vi "Location_Correction.vi"() -> ()   [LabVIEW 2017]
uses:
  <vilib>/Utility/file.llb/Write Delimited Spreadsheet (DBL).vi
  <vilib>/vision/driver/NI_Vision_Acquisition_Software.lvlib
  <vilib>/vision/NI_Vision_Development_Module.lvlib
panel:
  in  "OK Button":bool
  out "Boolean 2":bool
  out "X":dbl[](array[numeric])
  out "Boolean":bool
  out "Y":dbl[](array[numeric])
  out "選擇範圍 2":T1(plugin-control)
  out "error out":errorcluster
  in  "亮度":cluster{"Min":i32, "Max":i32}(slide)={"Min"=60, "Max"=157} scale=0.0..255.0
  in  "飽和度":cluster{"Min":i32, "Max":i32}(slide)={"Min"=0, "Max"=42} scale=0.0..255.0
  in  "色相":cluster{"Min":i32, "Max":i32}(slide)={"Min"=67, "Max"=120} scale=0.0..255.0
  out "顯示錯誤":errorcluster
  out "影像":T1(plugin-control)
  in  "stop":bool
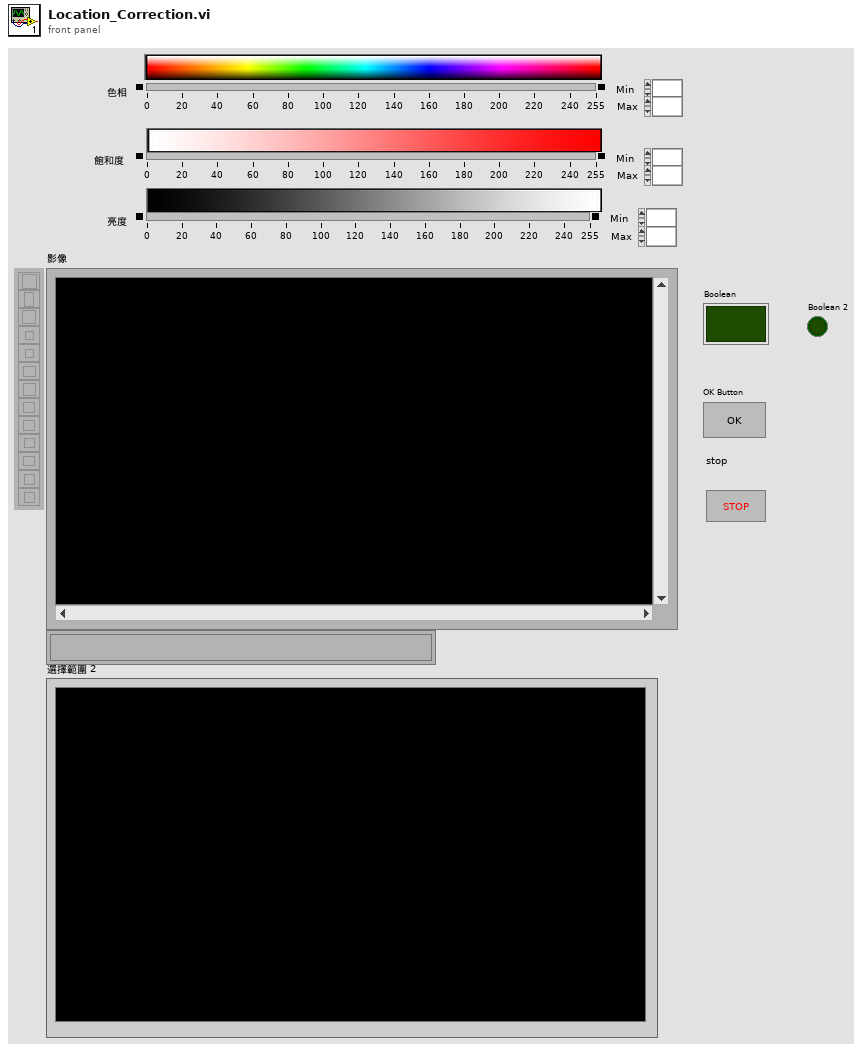
[diagram p1: front panel]
types:
  T1 = typedef "IMAQ Image.ctl" = refnum<image>
  T2 = typedef "Image Type" = u32
  T3 = cluster{"Type":u32, "Version":u32, "Flags":u32, "SerialNumberHigh":u32, "SerialNumberLow":u32, "BusType":u32, "InterfaceName":string, "VendorName":string, "ModelName":string, "CameraFileName":string, "CameraAttributeURL":string}[]
  T4 = cluster{"Type":u32, "Version":u32, "Flags":u32, "SerialNumberHigh":u32, "SerialNumberLow":u32, "BusType":u32, "InterfaceName":string, "VendorName":string, "ModelName":string, "CameraFileName":string, "CameraAttributeURL":string}
  T5 = typedef "IMAQdx.ctl" = refnum<k21>
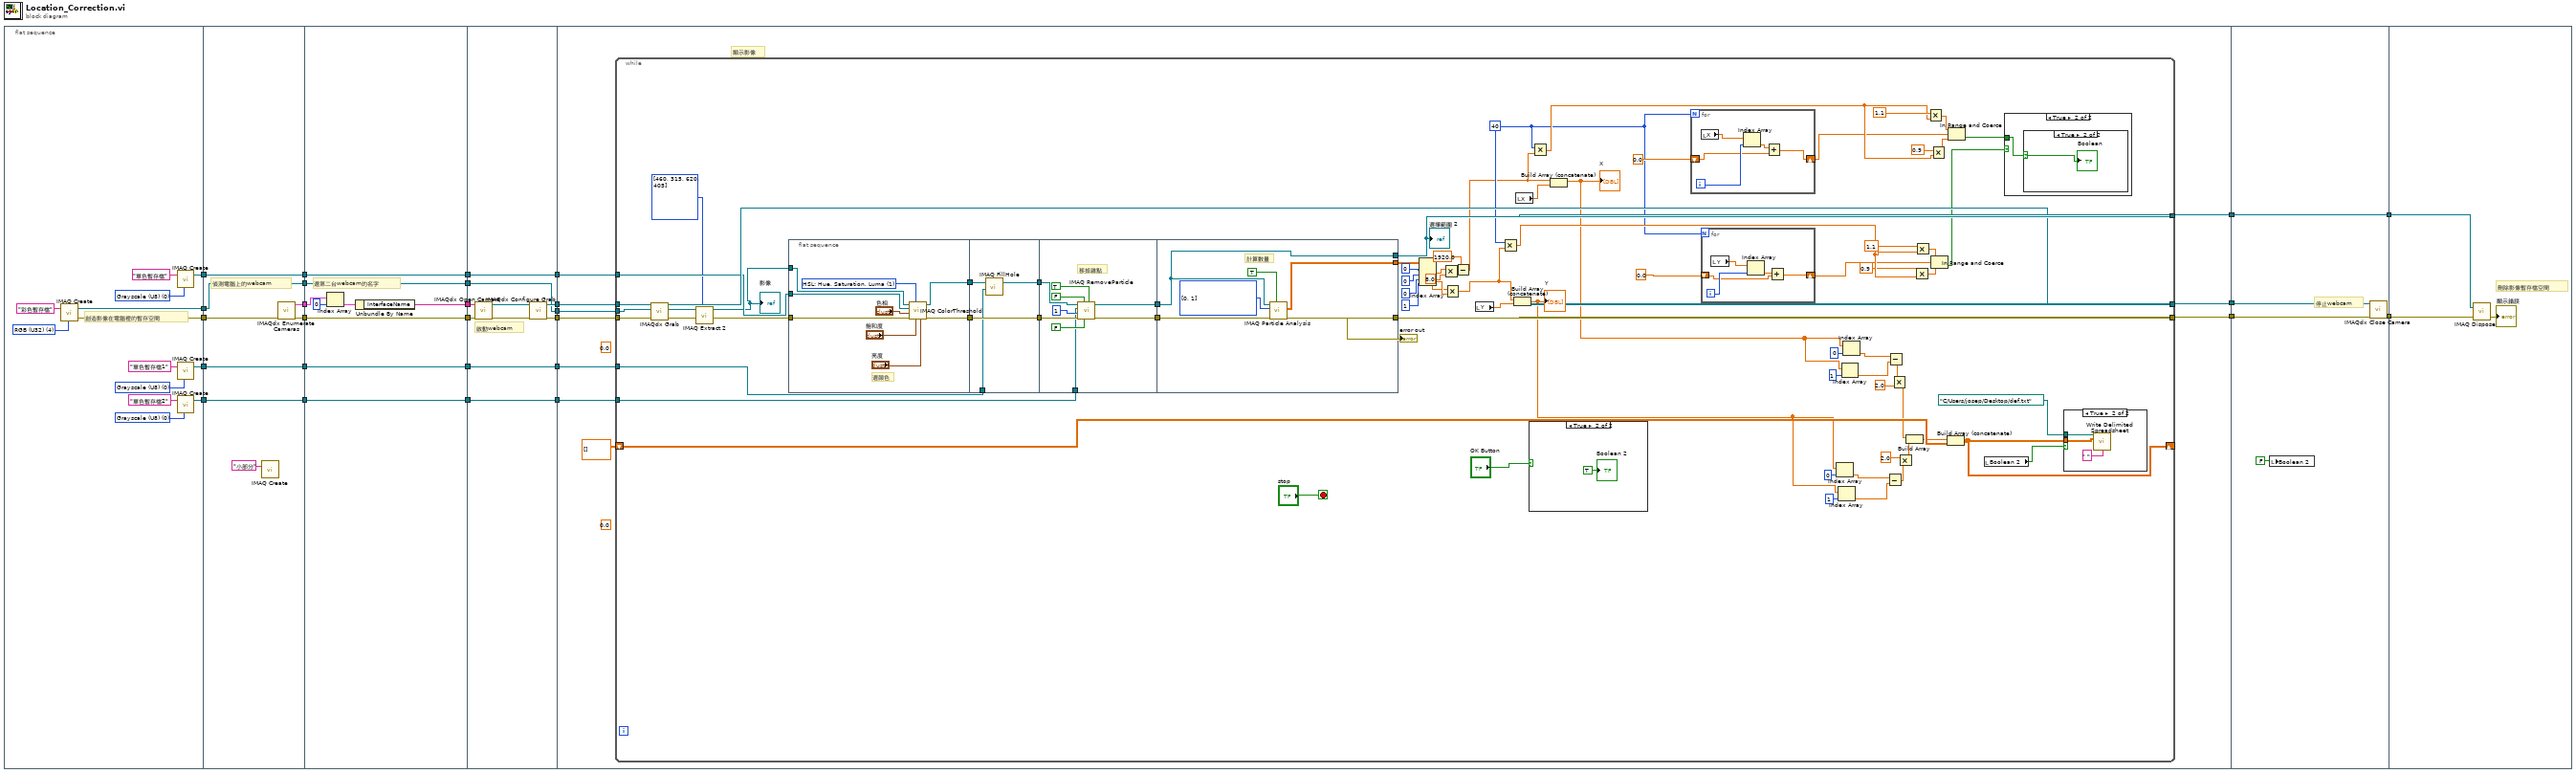
[diagram p0: block diagram]
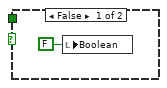
[diagram p4: hidden frame]
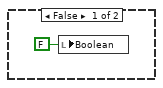
[diagram p5: hidden frame]
diagram:
  n1 = flat-sequence {
    tunnel: [w39] -> w22
    tunnel: [w38] -> w21
    tunnel: [w35] -> w12
    tunnel: [w30] -> w5
    tunnel: [w29] -> w1
    tunnel: [w49] -> w28
    tunnel: [w48] -> w23
    tunnel: w22 -> [w48]
    tunnel: w21 -> [w47]
    tunnel: [w46] -> w19
    tunnel: [w45] -> w13
    tunnel: w12 -> [w45]
    tunnel: [w44] -> w6
    tunnel: w5 -> [w44]
    tunnel: [w43] -> w2
    tunnel: w1 -> [w43]
    tunnel: w28 -> [w56]
    tunnel: [w55] -> w27
    tunnel: [w54] -> w24
    tunnel: w23 -> [w54]
    tunnel: [w53] -> w20
    tunnel: w19 -> [w53]
    tunnel: [w52] -> w14
    tunnel: w13 -> [w52]
    tunnel: [w51] -> w7
    tunnel: w6 -> [w51]
    tunnel: [w50] -> w3
    tunnel: w2 -> [w50]
    tunnel: w27 -> [w67]
    tunnel: [w66] -> w26
    tunnel: [w65] -> w25
    tunnel: w24 -> [w65]
    tunnel: w20 -> [w64]
    tunnel: [w62] -> w18
    tunnel: [w61] -> w15
    tunnel: w14 -> [w61]
    tunnel: [w60] -> w8
    tunnel: w7 -> [w60]
    tunnel: [w59] -> w4
    tunnel: w3 -> [w59]
    tunnel: w26 -> [w78]
    tunnel: w25 -> [w77]
    tunnel: w18 -> [w76]
    tunnel: [w75] -> w16
    tunnel: w15 -> [w74]
    tunnel: [w73] -> w11
    tunnel: [w72] -> w10
    tunnel: w8 -> [w71]
    tunnel: w4 -> [w70]
    tunnel: [w202] -> w17
    tunnel: w16 -> [w201]
    tunnel: w11 -> [w200]
    tunnel: w10 -> [w199]
    tunnel: [w199] -> w9
    tunnel: w17 -> [w205]
    tunnel: w9 -> [w203]
    frame #0 {
      w33 = T2 0 items=["Grayscale (U8)", "Grayscale (I16)", "Grayscale (SGL)", "Complex (CSG)", "RGB (U32)", "HSL (U32)", "RGB (U64)", "Grayscale (U16)"] ("Image Type")
      w34 = T2 0 items=["Grayscale (U8)", "Grayscale (I16)", "Grayscale (SGL)", "Complex (CSG)", "RGB (U32)", "HSL (U32)", "RGB (U64)", "Grayscale (U16)"] ("Image Type")
      w36 = T2 0 items=["Grayscale (U8)", "Grayscale (I16)", "Grayscale (SGL)", "Complex (CSG)", "RGB (U32)", "HSL (U32)", "RGB (U64)", "Grayscale (U16)"] ("Image Type")
      w41 = T2 4 items=["Grayscale (U8)", "Grayscale (I16)", "Grayscale (SGL)", "Complex (CSG)", "RGB (U32)", "HSL (U32)", "RGB (U64)", "Grayscale (U16)"] ("Image Type")
      # "創造影像在電腦裡的暫存空間"
      n2 = call "IMAQ Create"("Image Name"="彩色暫存檔", "Image Type"=w41) -> ("New Image"=w39:T1, "error out"=w38:errorcluster)  [unwired: 3 in]
      n3 = call "IMAQ Create"("Image Name"="單色暫存檔", "Image Type"=w36) -> ("New Image"=w35:T1)  [unwired: 3 in, 1 out]
      n4 = call "IMAQ Create"("Image Name"="單色暫存檔1", "Image Type"=w34) -> ("New Image"=w30:T1)  [unwired: 3 in, 1 out]
      n5 = call "IMAQ Create"("Image Name"="單色暫存檔2", "Image Type"=w33) -> ("New Image"=w29:T1)  [unwired: 3 in, 1 out]
    }
    frame #1 {
      # "偵測電腦上的webcam"
      n6 = call "IMAQ Create"("Image Name"="小部分") -> ()  [unwired: 4 in, 2 out]
      n7 = call <vilib>:"IMAQdx Enumerate Cameras.vi"("error in"=w47) -> ("error out"=w46:errorcluster, "Camera Information Array"=w49:T3)  [unwired: 9 in]
    }
    frame #2 {
      # "選第二台webcam的名字"
      n8 = Index Array(array=w56, index=0) -> (element=w57:T4)
      n9 = Unbundle By Name(w57) -> ("InterfaceName"=w55:string)
    }
    frame #3 {
      # "啟動webcam"
      n10 = call <vilib>:"IMAQdx Open Camera.vi"("error in"=w64, "Session In"=w67) -> ("error out"=w63:errorcluster, "Session Out"=w68:T5)  [unwired: 8 in]
      n11 = call <vilib>:"IMAQdx Configure Grab.vi"("error in"=w63, "Session In"=w68) -> ("error out"=w62:errorcluster, "Session Out"=w66:T5)  [unwired: 8 in]
    }
    frame #4 {
      (unwired) 0.0
      (unwired) 0.0
      # "顯示影像"
      n12 = while {
        tunnel: w78 -> [w150]
        tunnel: w77 -> [w110]
        tunnel: w76 -> [w149]
        tunnel: [w148] -> w75
        tunnel: w74 -> [w137]
        tunnel: [w139] -> w73
        tunnel: [w138] -> w72
        tunnel: w71 -> [w132]
        tunnel: w70 -> [w131]
        shift-right: [w97] -> _
        shift-left: dbl[][] [] -> [w98]
        stop <- "stop" stop-if-true
        w83 = 8.0 ("y")
        w106 = 40
        n13 = call <vilib>:"IMAQdx Grab.vi"("error in"=w149, "Image In"=w110, "Session In"=w150) -> ("error out"=w141:errorcluster, "Image Out"=w109:T1, "Session Out"=w148:T5)  [unwired: 5 in, 1 out]
        n14 = call "IMAQ Extract 2"("Optional Rectangle"=i32[] [460, 315, 620, 405], "Image Src"=w109) -> ("Image Dst Out"=w108:T1)  [unwired: 8 in, 1 out]
        "影像" <- w108
        n15 = flat-sequence {
          tunnel: w141 -> [w172]
          tunnel: w108 -> [w174]
          tunnel: [w171] -> w135
          tunnel: w137 -> [w173]
          tunnel: [w170] -> w133
          tunnel: [w180] -> w136
          tunnel: w135 -> [w182]
          tunnel: [w182] -> w134
          tunnel: w133 -> [w181]
          tunnel: w132 -> [w179]
          tunnel: [w185] -> w143
          tunnel: [w184] -> w142
          tunnel: w136 -> [w187]
          tunnel: w134 -> [w186]
          tunnel: w131 -> [w183]
          tunnel: [w196] -> w138
          tunnel: [w192] -> w139
          tunnel: w143 -> [w195]
          tunnel: w142 -> [w196]
          tunnel: [w193] -> w140
          frame #0 {
            w175 = 1 items=["RGB (Red, Green, Blue)", "HSL: Hue, Saturation, Luma"] ("Threshold Color Mode")
            # "選顏色"
            n16 = call "IMAQ ColorThreshold"("Blue or Luma or Val or Inten Range"="亮度", "Green or Sat Range"="飽和度", "Color Mode"=w175, "error in (no error)"=w172, "Red or Hue Range"="色相", "Image Dst"=w173, "Image Src"=w174) -> ("error out"=w171:errorcluster, "Image Dst Out"=w170:T1)  [unwired: 1 in, 2 out]
          }
          frame #1 {
            n17 = call "IMAQ FillHole"("Image Dst"=w179, "Image Src"=w181) -> ("Image Dst Out"=w180:T1)  [unwired: 2 in, 3 out]
          }
          frame #2 {
            # "移掉雜點"
            n18 = call "IMAQ RemoveParticle"("Connectivity 4/8 (8)"=TRUE, "Low Pass/High Pass (Low)"=FALSE, "Square/Hexa (Square)"=FALSE, "error in (no error)"=w186, "Number of Erosion"=1, "Image Dst"=w183, "Image Src"=w187) -> ("error out"=w185:errorcluster, "Image Dst Out"=w184:T1)  [unwired: 3 out]
          }
          frame #3 {
            w194 = i32[] [0, 1] items=["Center of Mass X", "Center of Mass Y", "First Pixel X", "First Pixel Y", "Bounding Rect Left", "Bounding Rect Top", "Bounding Rect Right", "Bounding Rect Bottom", "Max Feret Diameter Start X", "Max Feret Diameter Start Y", "Max Feret Diameter End X", "Max Feret Diameter End Y", "Max Horiz. Segment Length Left", "Max Horiz. Segment Length Right", "Max Horiz. Segment Length Row", "-", "Bounding Rect Width", "Bounding Rect Height", "Bounding Rect Diagonal", "Perimeter", "Convex Hull Perimeter", "Holes' Perimeter", "Max Feret Diameter", "Equivalent Ellipse Major Axis", "Equivalent Ellipse Minor Axis", "Equivalent Ellipse Minor Axis (Feret)", "Equivalent Rect Long Side", "Equivalent Rect Short Side", "Equivalent Rect Diagonal", "Equivalent Rect Short Side (Feret)", "Average Horiz. Segment Length", "Average Vert. Segment Length", "Hydraulic Radius", "Waddel Disk Diameter", "-", "Area", "Holes' Area", "Particle & Holes' Area", "Convex Hull Area", "Image Area", "-", "Number of Holes", "Number of Horiz. Segments", "Number of Vert. Segments", "-", "Orientation", "Max Feret Diameter Orientation", "-", "% Area/Image Area", "% Area/(Particle & Holes' Area)", "Ratio of Equivalent Ellipse Axes", "Ratio of Equivalent Rect Sides", "-", "Elongation Factor", "Compactness Factor", "Heywood Circularity Factor", "Type Factor", "-", "Sum X", "Sum Y", "Sum XX", "Sum XY", "Sum YY", "Sum XXX", "Sum XXY", "Sum XYY", "Sum YYY", "-", "Moment of Inertia XX", "Moment of Inertia XY", "Moment of Inertia YY", "Moment of Inertia XXX", "Moment of Inertia XXY", "Moment of Inertia XYY", "Moment of Inertia YYY", "Norm. Moment of Inertia XX", "Norm. Moment of Inertia XY", "Norm. Moment of Inertia YY", "Norm. Moment of Inertia XXX", "Norm. Moment of Inertia XXY", "Norm. Moment of Inertia XYY", "Norm. Moment of Inertia YYY", "Hu Moment 1", "Hu Moment 2", "Hu Moment 3", "Hu Moment 4", "Hu Moment 5", "Hu Moment 6", "Hu Moment 7"] ("Pixel Measurements")
            # "計算數量"
            n19 = call "IMAQ Particle Analysis"("Connectivity 4/8 (8)"=TRUE, "error in (no error)"=w195, "Pixel Measurements"=w194, "Image"=w196) -> ("error out"=w192:errorcluster, "Particle Measurements (Pixels)"=w193:dbl[][])  [unwired: 1 in, 5 out]
          }
        }
        n20 = Index Array(array=w140, index (row) #1=0 ("disabled index (row)"), index (col) #1=0 ("disabled index (col)"), index (row) #2=0 ("index (row)"), index (col) #2=1 ("disabled index (col)")) -> (element #1=w120:dbl, element #2=w122:dbl)
        n21 = Multiply(x=w120, y=w83) -> (x*y=w105:dbl)
        n22 = Multiply(x=w83, y=w122) -> (x*y=w101:dbl)
        n23 = Subtract(x=1920.0, y=w105) -> (x-y=w102:dbl)
        n24 = local read "Y"() -> (w130:dbl[])
        n25 = Multiply(x=w106, y=w101) -> (x*y=w126:dbl)
        n26 = Build Array (concatenate)(w101, w130) -> (w91:dbl[])
        "Y" <- w91
        n27 = local read "X"() -> (w121:dbl[])
        n28 = case shown="True" "OK Button" {
          frame False {
          }
          frame True {
            "Boolean 2" <- TRUE ("Boolean 2")
          }
        }
        n29 = Multiply(x=w106, y=w102) -> (x*y=w114:dbl)
        n30 = Build Array (concatenate)(w102, w121) -> (w92:dbl[])
        "X" <- w92
        n31 = for {
          N: w106 -> [_]
          shift-right: [w161] -> w113
          shift-left: 0.0 -> [w160]
          i -> [w163]
          n32 = local read "X"() -> (w164:dbl[])
          n33 = Index Array(array=w164, index=w163) -> (element=w162:dbl)
          n34 = Add(x=w162, y=w160) -> (x+y=w161:dbl)
        }
        n35 = for {
          N: w106 -> [_]
          shift-right: [w166] -> w125
          shift-left: 0.0 -> [w165]
          i -> [w168]
          n36 = local read "Y"() -> (w169:dbl[])
          n37 = Index Array(array=w169, index=w168) -> (element=w167:dbl)
          n38 = Add(x=w167, y=w165) -> (x+y=w166:dbl)
        }
        n39 = Index Array(array=w91, index=0) -> (element=w87:dbl)
        n40 = Index Array(array=w91, index=1) -> (element=w86:dbl)
        n41 = Index Array(array=w92, index=1) -> (element=w89:dbl)
        n42 = Index Array(array=w92, index=0) -> (element=w90:dbl)
        n43 = Subtract(x=w87, y=w86) -> (x-y=w85:dbl)
        n44 = Subtract(x=w90, y=w89) -> (x-y=w88:dbl)
        n45 = Multiply(x=w88, y=2.0) -> (x*y=w82:dbl)
        n46 = Multiply(x=2.0, y=w85) -> (x*y=w80:dbl)
        n47 = Build Array(w82, w80) -> (w84:dbl[])
        n48 = Multiply(x=0.9, y=w126) -> (x*y=w127:dbl)
        n49 = Multiply(x=1.1, y=w126) -> (x*y=w128:dbl)
        n50 = Multiply(x=1.1, y=w114) -> (x*y=w118:dbl)
        n51 = Multiply(x=0.9, y=w114) -> (x*y=w117:dbl)
        n52 = In Range and Coerce(upper limit=w128, x=w125, lower limit=w127) -> (In Range?=w112:bool)  [unwired: 1 out]
        n53 = Build Array (concatenate)(w84, w98) -> (w97:dbl[][])
        n54 = In Range and Coerce(upper limit=w118, x=w113, lower limit=w117) -> (In Range?=w111:bool)  [unwired: 1 out]
        n55 = local read "Boolean 2"() -> (w99:bool)
        n56 = case shown="True" w112 {
          tunnel: w111 -> [_ w157]
          frame False {
            n57 = local write "Boolean"(FALSE ("Boolean")) -> ()
          }
          frame True {
            n58 = case shown="True" w157 {
              selector: w157 -> [_ w159]
              frame False {
                n59 = local write "Boolean"(FALSE ("Boolean")) -> ()
              }
              frame True {
                "Boolean" <- w159
              }
            }
          }
        }
        n60 = case shown="True" w99 {
          tunnel: path "C:/Users/josep/Desktop/def.txt" ("file path (dialog if empty)") -> [_ w154]
          tunnel: w97 -> [_ w153]
          frame False {
          }
          frame True {
            n61 = call-poly <vilib>:"Write Delimited Spreadsheet.vi"("file path (dialog if empty)"=w154, "2D data"=w153, "delimiter (\\t)"=" " ("delimiter (\\t)")) -> ()  [unwired: 11 in, 2 out]
          }
        }
        "error out" <- w139
        "選擇範圍 2" <- w138
      }
    }
    frame #5 {
      # "停止webcam"
      n62 = local write "Boolean 2"(FALSE ("Boolean 2")) -> ()
      n63 = call <vilib>:"IMAQdx Close Camera.vi"("error in"=w200, "Session In"=w201) -> ("error out"=w202:errorcluster)  [unwired: 9 in]
    }
    frame #6 {
      # "刪除影像暫存檔空間"
      n64 = call "IMAQ Dispose"("Image"=w203, "error in (no error)"=w205) -> ("error out"=→"顯示錯誤":errorcluster)  [unwired: 4 in]
    }
  }
